vi "Drive_Execute.vi"   [LabVIEW 2019]
uses:
  Utility_VIs/Basic_Motor_Modes.ctl
  Drive_Globals.vi
  <vilib>/Rock Robotics/WPI/Joystick/WPI_JoystickArcadeMapping.vi
types:
  T1 = typedef "Basic_Motor_Modes.ctl" = enum16{"Percent_Voltage", "Speed_Control", "Position_Control", "Current"}
  T2 = typedef "Drive_Cluster.ctl" = cluster{"Control_State":T3, "Angular_Throttle":dbl, "Linear_Throttle":dbl, "Torque_Changing":bool, "Step":dbl, "Parameter_1":dbl, "Parameter_2":dbl, "Parameter_3":dbl, "Parameter_4":dbl, "Auto_Notifier":refnum<notifier>}
  T3 = typedef "Drive_States.ctl" = enum16{"Percent_Voltage_Control", "Speed_Control", "Command_HeadingDistance", "Command_TurnToHeading", "Command_FollowPath"}
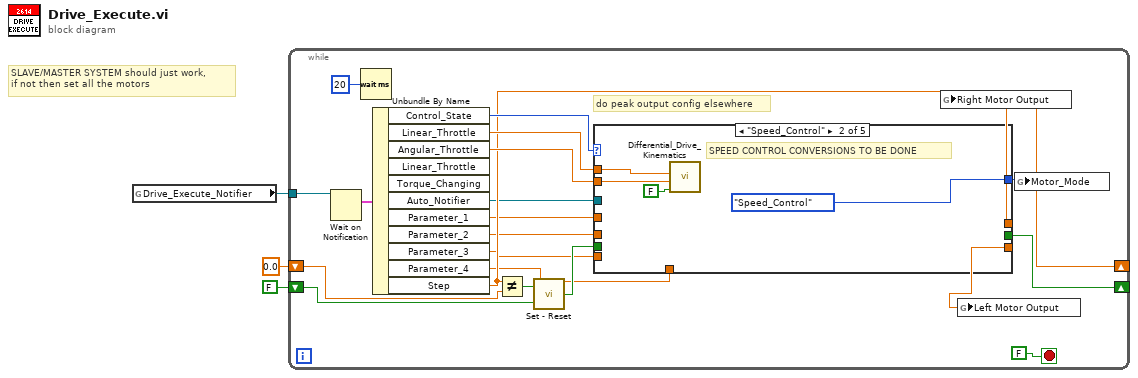
[diagram p0: block diagram]
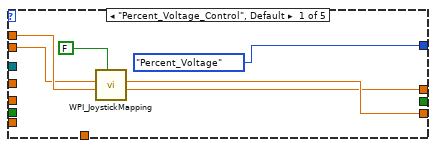
[diagram p2: hidden frame]
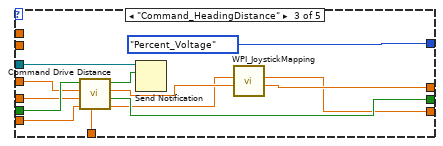
[diagram p3: hidden frame]
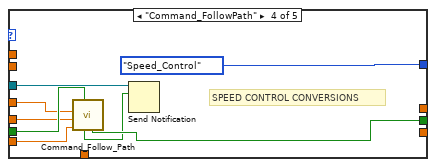
[diagram p4: hidden frame]
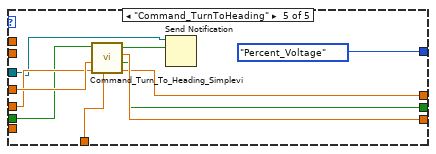
[diagram p5: hidden frame]
diagram:
  # "SLAVE/MASTER SYSTEM should just work, \nif not then set all the motors"
  n1 = global read "Drive_Globals.vi" "Drive_Execute_Notifier"() -> (w3:refnum<notifier>)
  n2 = while {
    tunnel: w3 -> [w24]
    shift-right: [w11] -> _
    shift-left: FALSE ("Square Inputs") -> [w14]
    shift-right: [w17] -> _
    shift-left: 0.0 ("Step") -> [w16]
    stop <- FALSE stop-if-true
    # "do peak output config elsewhere"
    n3 = Wait on Notification(notifier=w24) -> (notification=w23:T2)  [unwired: 3 in, 3 out]
    n4 = Wait (ms)(milliseconds to wait=u32 20) -> ()  [unwired: 1 out]
    n5 = Unbundle By Name(w23) -> ("Control_State"=w22:T3, "Linear_Throttle"=w20:dbl, "Angular_Throttle"=w19:dbl, "Auto_Notifier"=w12:refnum<notifier>, "Parameter_1"=w10:dbl, "Parameter_2"=w9:dbl, "Parameter_3"=w8:dbl, "Parameter_4"=w7:dbl, "Step"=w17:dbl)  [unwired: 2 out]
    n6 = Not Equal?(x=w17, y=w16) -> (x != y?=w15:bool)
    n7 = call "Set - Reset.vi"("Reset"=w14, "Set"=w15) -> ("Output"=w13:bool)
    n8 = case shown="\"Speed_Control\"" w22 {
      tunnel: w20 -> [w30 w33 _ _ _]
      tunnel: w19 -> [w29 w32 _ _ _]
      tunnel: [w28 _ w36 _ w61] -> w6
      tunnel: [w27 _ w37 _ w60] -> w5
      tunnel: w13 -> [_ _ w45 w53 w62]
      tunnel: w12 -> [_ _ w47 w55 w58]
      tunnel: [_ _ w46 w54 w59] -> w11
      tunnel: w10 -> [_ _ w44 w52 w65]
      tunnel: w9 -> [_ _ w43 w51 w64]
      tunnel: w8 -> [_ _ w41 w49 _]
      tunnel: w7 -> [_ _ w40 _ w63]
      tunnel: [Basic_Motor_Modes."Percent_Voltage" ("Basic_Motor_Mode") Basic_Motor_Modes."Speed_Control" ("Basic_Motor_Mode") Basic_Motor_Modes."Percent_Voltage" ("Basic_Motor_Mode") Basic_Motor_Modes."Speed_Control" ("Basic_Motor_Mode") Basic_Motor_Modes."Percent_Voltage" ("Basic_Motor_Mode")] -> w4
      frame "Percent_Voltage_Control", Default {
        n9 = call-poly <vilib>:"WPI_JoystickMapping.vi"("Square Inputs"=FALSE, "Y axis value"=w30, "X axis value"=w29) -> ("Right Motor Value"=w27:dbl, "Left Motor Value"=w28:dbl)  [unwired: 7 in]
      }
      frame "Speed_Control" {
        # "SPEED CONTROL CONVERSIONS TO BE DONE"
        n10 = call "Differential_Drive_Kinematics.vi"("Scale_Down_For_Turn"=FALSE, "Angular_Throttle"=w32, "Linear_Throttle"=w33) -> ()  [unwired: 7 in, 2 out]
      }
      frame "Command_HeadingDistance" {
        n11 = call "Command Drive Distance.vi"("Timeout"=w40, "Speed"=w41, "Heading"=w43, "Distance(Feet)"=w44, "Startup"=w45) -> ("Angular"=w38:dbl, "Reinit"=w46:bool, "Linear"=w39:dbl, "Completed"=w42:bool)  [unwired: 3 in]
        n12 = Send Notification(notification=w42, notifier=w47) -> ()  [unwired: 1 in, 2 out]
        n13 = call-poly <vilib>:"WPI_JoystickMapping.vi"("Y axis value"=w39, "X axis value"=w38) -> ("Right Motor Value"=w37:dbl, "Left Motor Value"=w36:dbl)  [unwired: 8 in]
      }
      frame "Command_FollowPath" {
        # "SPEED CONTROL CONVERSIONS"
        n14 = call "Command_Follow_Path.vi"("Startup"=w53, "timeout"=w49, "acceptable angle error"=w51, "acceptable distance error"=w52) -> ("Reint"=w54:bool, "Completed"=w50:bool)  [unwired: 4 in, 2 out]
        n15 = Send Notification(notification=w50, notifier=w55) -> ()  [unwired: 1 in, 2 out]
      }
      frame "Command_TurnToHeading" {
        n16 = call "Command_Turn_To_Heading_Simplevi.vi"("Timeout"=w63, "Speed"=w64, "Heading"=w65, "Startup"=w62) -> ("Right Wheel"=w60:dbl, "Reinit"=w59:bool, "Left Wheel"=w61:dbl, "Completed"=w57:bool)  [unwired: 4 in]
        n17 = Send Notification(notification=w57, notifier=w58) -> ()  [unwired: 1 in, 2 out]
      }
    }
    n18 = global write "Drive_Globals.vi" "Right Motor Output"(w5) -> ()
    n19 = global write "Drive_Globals.vi" "Left Motor Output"(w6) -> ()
    n20 = global write "Drive_Globals.vi" "Motor_Mode"(w4) -> ()
  }
